vi "Close Hardware.vi"(8 "error in (no error)":errorcluster, 11 "Instrument.Template in":refnum<class "Instrument.LN2.lvclass">) -> (0 "error out":errorcluster, 3 "Instrument.Template out":refnum<class "Instrument.LN2.lvclass">)   [LabVIEW 2019, in "Instrument.LN2.lvclass"]
uses:
  Instrument.LN2.lvclass
  Instrument.LN2.lvclass/Instrument.LN2.ctl
  <userlib>/LevyLab/Instrument Framework/Instrument Types/VSource/Instrument.VSource.lvclass
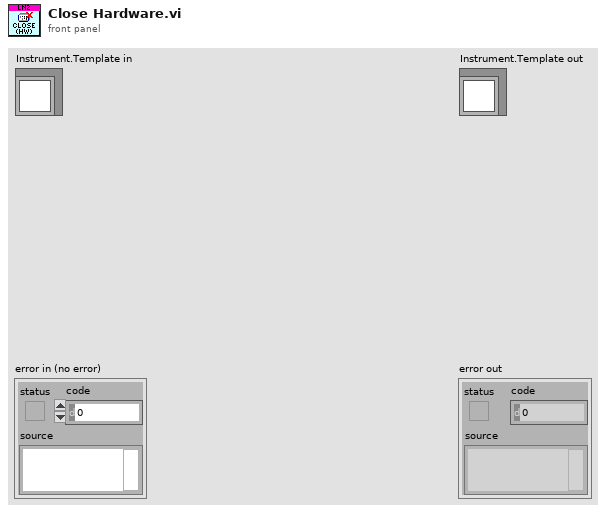
[diagram p1: front panel]
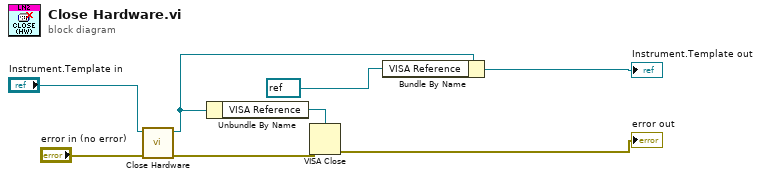
[diagram p0: block diagram]
diagram:
  n1 = call-parent "Close Hardware.vi"("error in (no error)"="error in (no error)", "Instrument in"="Instrument.Template in") -> ("error out"=w6:errorcluster, "Instrument out"=w3:refnum<class "Instrument.LN2.lvclass">)  [unwired: 8 in]
  n2 = Unbundle By Name(w3) -> ("VISA Reference"=w5:refnum<visa-resource-name>)
  n3 = VISA Close(VISA resource name=w5, error in (no error)=w6) -> (error out=→"error out":errorcluster)
  n4 = Bundle By Name(cluster=w3, "VISA Reference"=refnum<visa-resource-name> refnum) -> (→"Instrument.Template out":refnum<class "Instrument.LN2.lvclass">)
